vi "createMissionWaypoints.vi"(8 "error in (no error)":errorcluster, 11 "Drive in":refnum<class "DriveTo.lvclass">) -> (0 "error out":errorcluster, 3 "Drive out":refnum<class "DriveTo.lvclass">)   [LabVIEW 2011, in "DriveTo.lvclass"]
uses:
  DriveTo.lvclass
  DriveTo.lvclass/DriveTo.ctl
  2 Globals/2 Global.vi
  Waypoint/Waypoint.lvclass
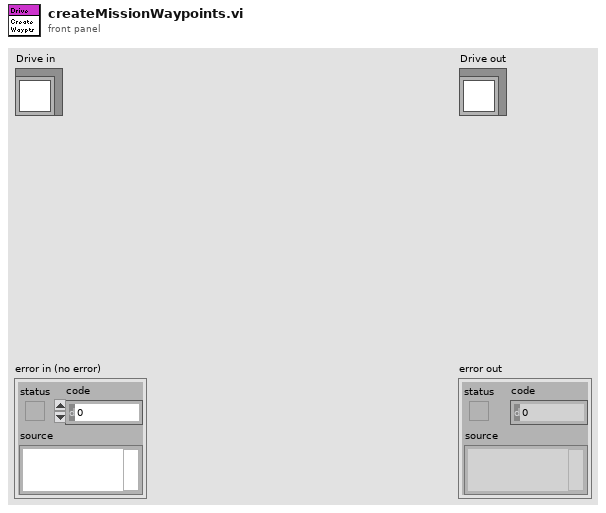
[diagram p1: front panel]
types:
  T1 = typedef "UTM Location.ctl" = cluster{"UTM Zone":dbl, "Hemisphere":enum16{"North", "South"}, "East":dbl, "North":dbl}
  T2 = typedef "Waypoints List.ctl" = refnum<class "Waypoint.lvclass">[]
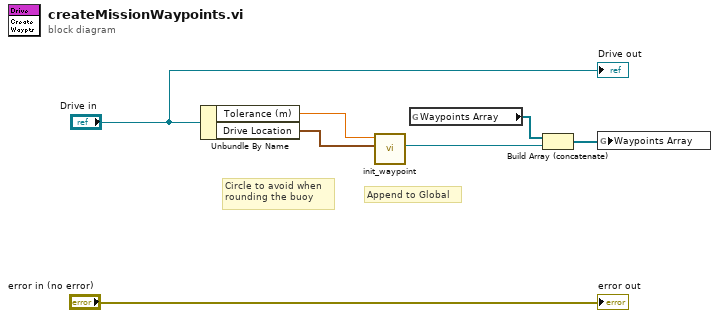
[diagram p0: block diagram]
diagram:
  # "Append to Global"
  # "Circle to avoid when\nrounding the buoy"
  n1 = Unbundle By Name("Drive in") -> ("Tolerance (m)"=w7:dbl, "Drive Location"=w6:T1)
  n2 = call "init_waypoint.vi"("Coords"=w6, "Tolerance (m)"=w7) -> ("Waypoint Out"=w3:refnum<class "Waypoint.lvclass">)  [unwired: 9 in]
  n3 = global read "2 Global.vi" "Waypoints Array"() -> (w5:T2)
  n4 = Build Array (concatenate)(w5, w3) -> (w4:T2)
  n5 = global write "2 Global.vi" "Waypoints Array"(w4) -> ()
  "error out" <- "error in (no error)"
  "Drive out" <- "Drive in"
